vi "Extract Ethernet Protocol.vi"() -> ()   [LabVIEW 2025]
panel:
  out "PROTOCOL":T1
  in  "value":T2
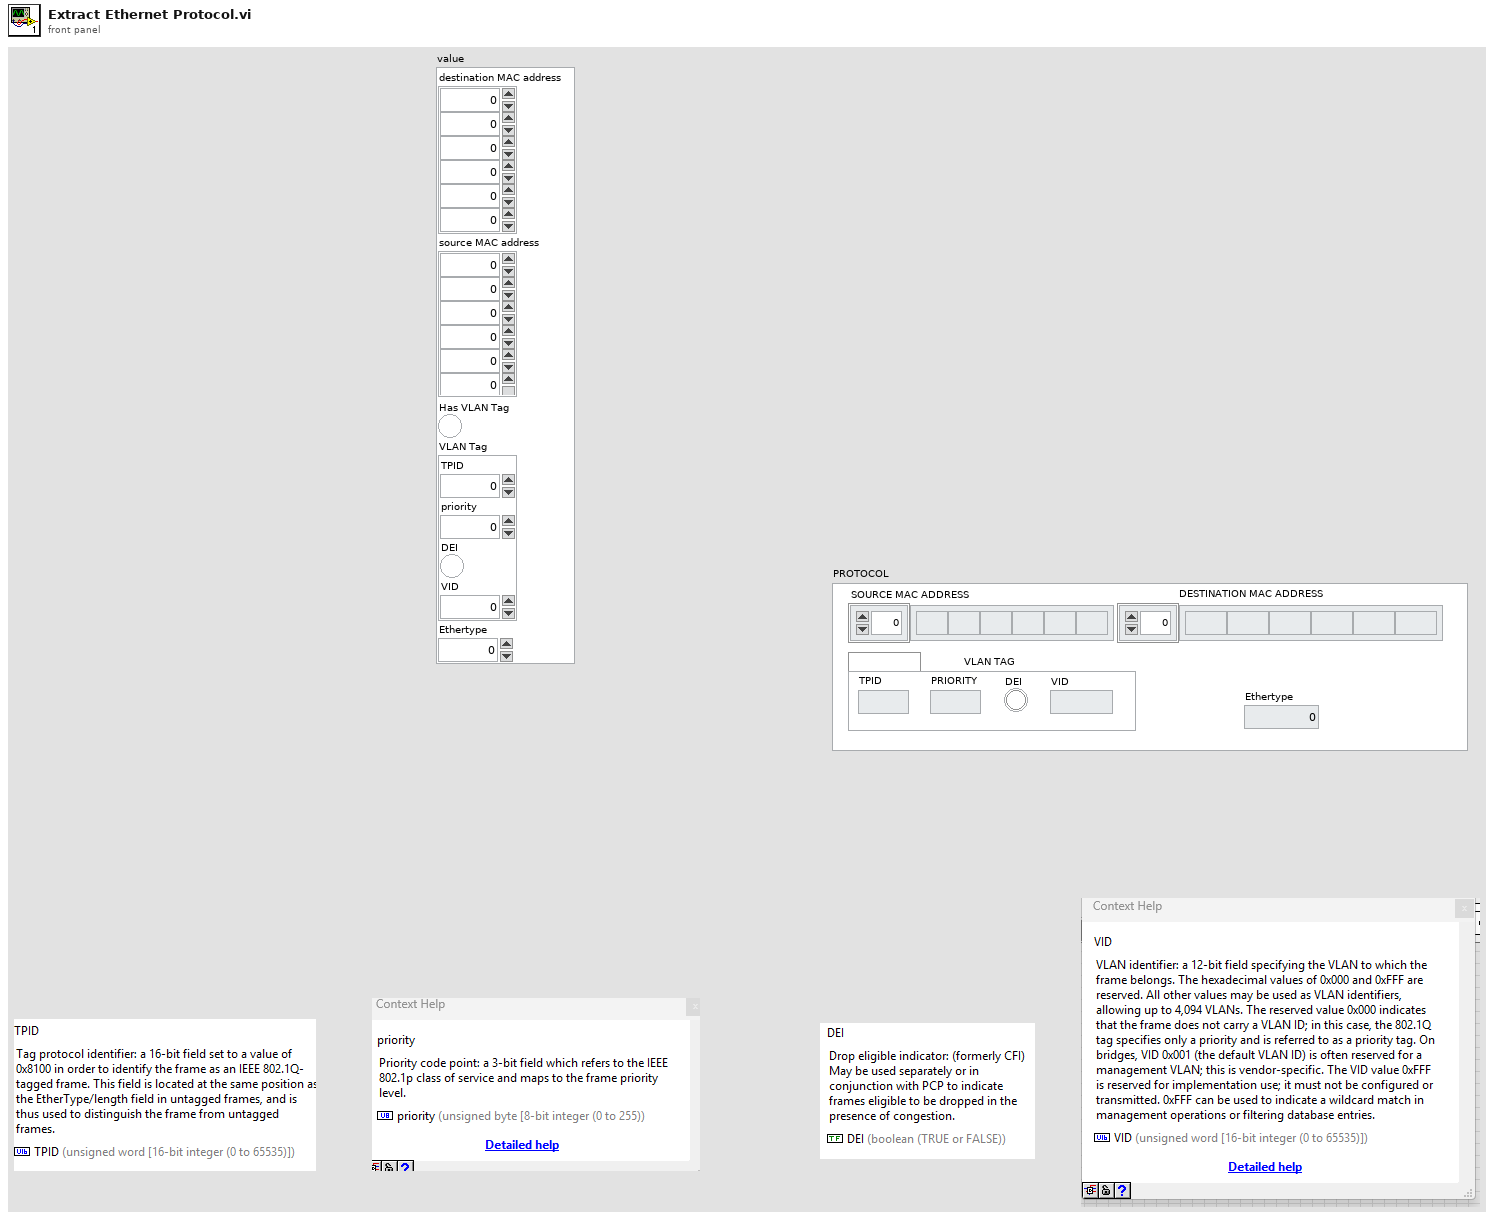
[diagram p1: front panel]
types:
  T1 = cluster{"SOURCE MAC ADDRESS":u8[], "DESTINATION MAC ADDRESS":u8[], "Has VLAN":bool, "VLAN TAG":cluster{"TPID":u16, "PRIORITY":u8, "DEI":bool, "VID":u16}, "Ethertype":u16}
  T2 = cluster{"destination MAC address":cluster{"Numeric":u8, "Numeric":u8, "Numeric":u8, "Numeric":u8, "Numeric":u8, "Numeric":u8}, "source MAC address":cluster{"Numeric":u8, "Numeric":u8, "Numeric":u8, "Numeric":u8, "Numeric":u8, "Numeric":u8}, "Has VLAN Tag":bool, "VLAN Tag":cluster{"TPID":u16, "priority":u8, "DEI":bool, "VID":u16}, "Ethertype":u16}
  T3 = cluster{"Numeric":u8, "Numeric":u8, "Numeric":u8, "Numeric":u8, "Numeric":u8, "Numeric":u8}
  T4 = cluster{"TPID":u16, "priority":u8, "DEI":bool, "VID":u16}
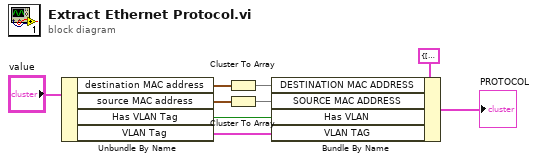
[diagram p0: block diagram]
diagram:
  n1 = Unbundle By Name("value") -> ("destination MAC address"=w8:T3, "source MAC address"=w6:T3, "Has VLAN Tag"=w3:bool, "VLAN Tag"=w2:T4)
  n2 = Cluster To Array(cluster=w8) -> (array=w7:u8[])
  n3 = Cluster To Array(cluster=w6) -> (array=w5:u8[])
  n4 = Bundle By Name(cluster=T1 {"SOURCE MAC ADDRESS"=[0, 7, 0, 0, 0, 0], "DESTINATION MAC ADDRESS"=[0, 0, 0, 0, 0, 0], "Has VLAN"=FALSE, "VLAN TAG"={"TPID"=0, "PRIORITY"=0, "DEI"=FALSE, "VID"=0}, "Ethertype"=0} ("Cluster 3"), "DESTINATION MAC ADDRESS"=w7, "SOURCE MAC ADDRESS"=w5, "Has VLAN"=w3, "VLAN TAG"=w2) -> (→"PROTOCOL":T1)
